vi "Get IO Direction.vi"(8 "error in (no error)":errorcluster, 10 "iDirection":i32, 11 "index":i32) -> (0 "error out":errorcluster, 2 "iDirection out":i32, 3 "function return":u32)   [LabVIEW 2014, in "atmcd32d.lvlib"]
doc: "unsigned int WINAPI GetIODirection(int index, int * iDirection);"
uses:
  atmcd32d.lvlib
  atmcd32d.dll
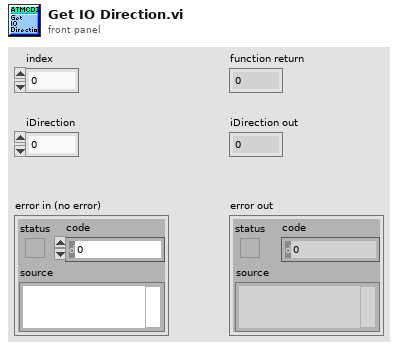
[diagram p1: front panel]
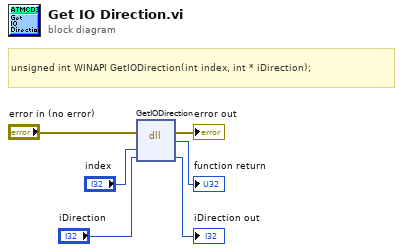
[diagram p0: block diagram]
diagram:
  # "unsigned int WINAPI GetIODirection(int index, int * iDirection);"
  n1 = dll-call lib="C:/Users/Bakir/Documents/Lambda2-Testing/lib/Andorlib/atmcd32d.*" fn="GetIODirection"(error in="error in (no error)", "index"="index", "iDirection"="iDirection") -> (error out=→"error out":errorcluster, →"function return":u32, "iDirection"=→"iDirection out":i32)  [unwired: 3 in, 1 out]
